vi "Pointer producer consumer Read Voltage.vi"(7 "Total Stop":bool, 8 "error in (no error)":errorcluster, 9 "Speed":u8, 10 "Diodes ON/OFF":bool=TRUE, 11 "Data in":T1={"[V]"=0.0, "Vertical sum"=0.0, "Horizontal sum"=0.0, "auto Loopback"=FALSE, "Auto Balance"=FALSE, "Out Cmd"=0, "Motor Cmd"=0, "ADC Values"=[], "Clouds ctrl"=FALSE, "Cloud Det"=FALSE, "Cloud Sens"=0, "Loops"=0, "VISA res"="COM3"} {"Motor Cmd" format="%x"}) -> (0 "Diods cable OFF status":bool, 1 "Diods cable OFF status request":bool, 2 "ADC votlages":dbl[](array[numeric]), 4 "error out":errorcluster, 5 "Motor Cmd":string=" ")   [LabVIEW 2014]
doc: "INPUTS - baud rate & VISA resource name & convertor selector & motor controler\n\nThis VI sends short HEX number to ATMEGA8 via USB-serial port by NI, and then transform read HEX number into values of convertor Voltage. \n\nOUTPUTS - voltage from ADC0, ADC1, ADC2, ADC3 in ATMEGA8"
uses:
  Ctrls/Data cluster.ctl
panel:
  out "Alfa limit switch":bool
  out "Voltage on ADC0 - UP":dbl format="%#_4g"
  out "Voltage on ADC3 - RIGHT":dbl format="%#_4g"
  out "Voltage on ADC1 - LEFT":dbl format="%#_4g"
  out "Voltage on ADC2 - DOWN":dbl format="%#_4g"
  out "Serial output":string
  out "Serial input":string=" "
  out "VISA resource name":refnum<visa-resource-name>="COM3"
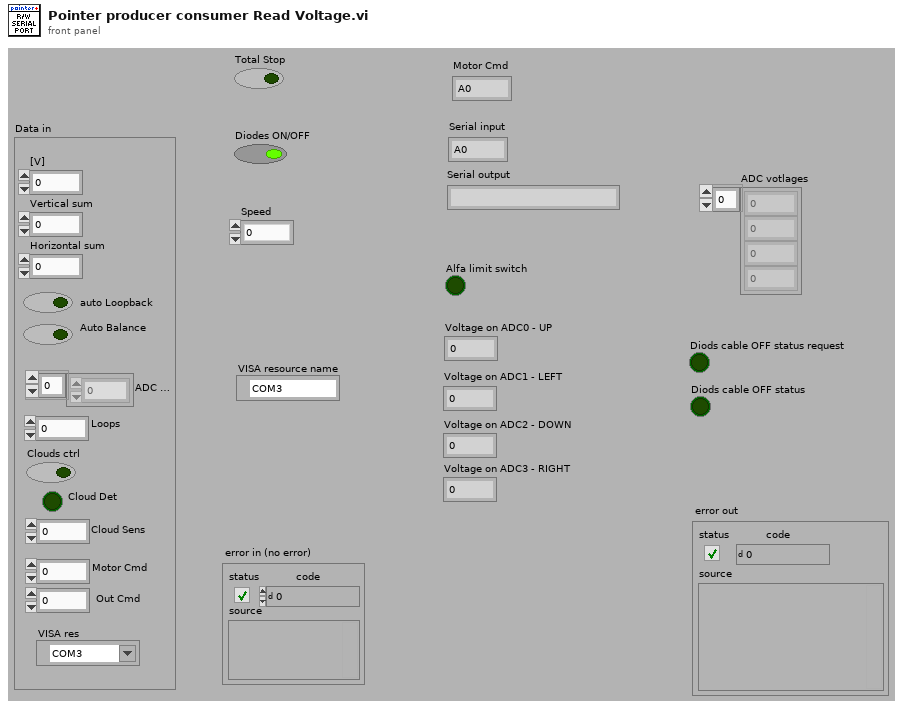
[diagram p1: front panel]
types:
  T1 = typedef "Data cluster.ctl" = cluster{"[V]":dbl, "Vertical sum":dbl, "Horizontal sum":dbl, "auto Loopback":bool, "Auto Balance":bool, "Out Cmd":i32, "Motor Cmd":i32, "ADC Values":dbl[], "Clouds ctrl":bool, "Cloud Det":bool, "Cloud Sens":i8, "Loops":u8, "VISA res":refnum<visa-resource-name>}
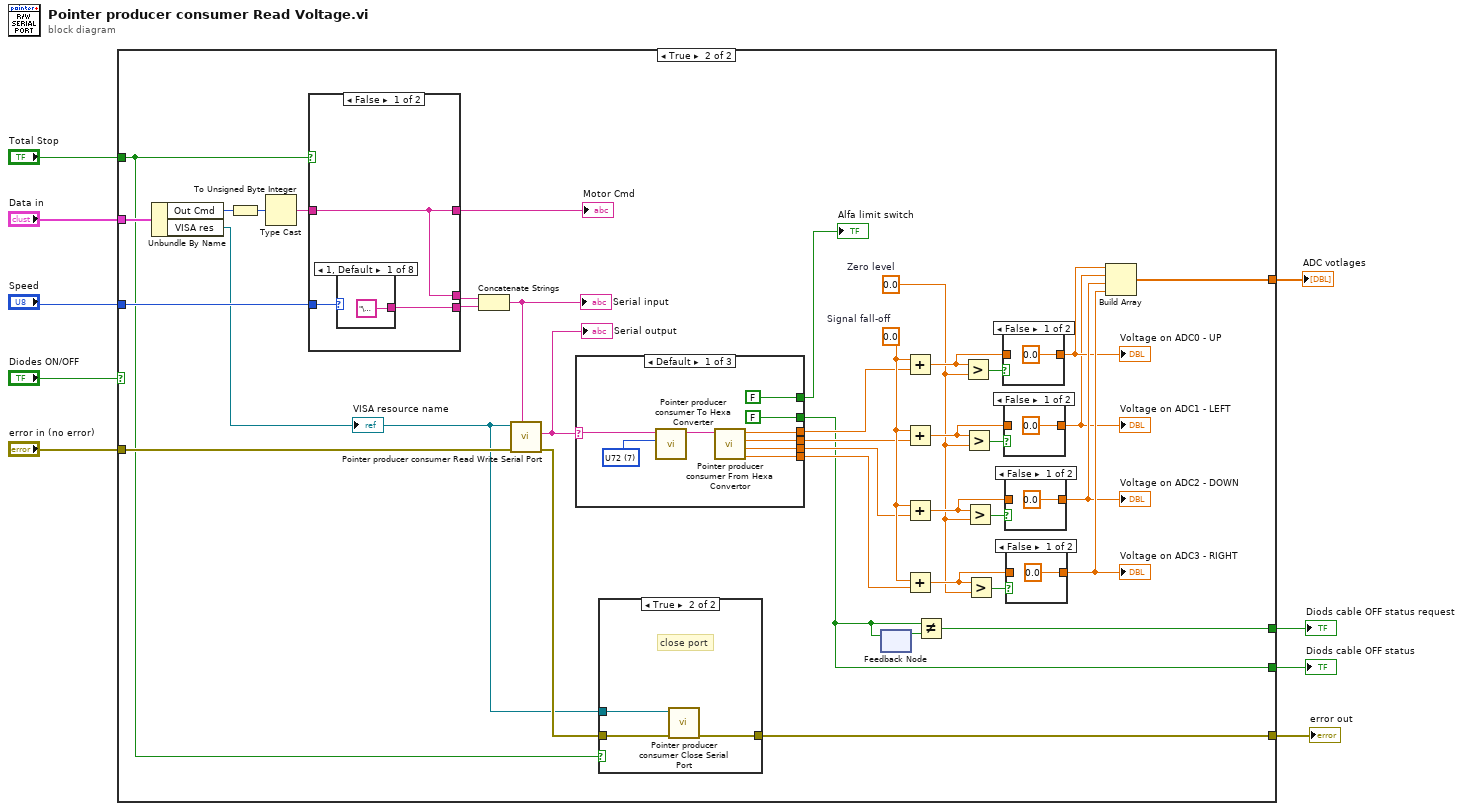
[diagram p0: block diagram]
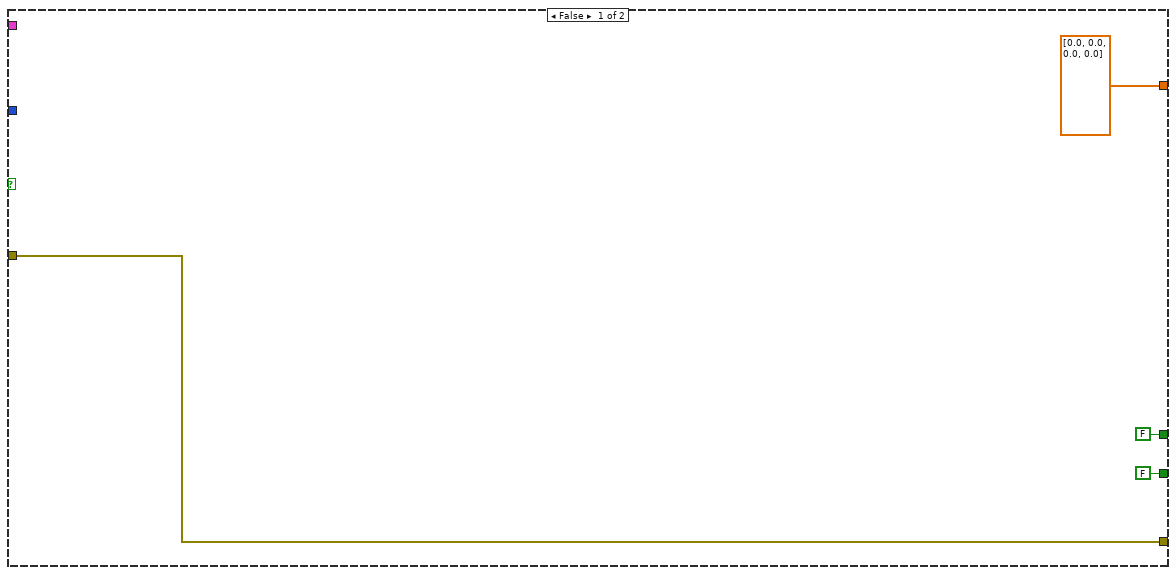
[diagram p2: hidden frame]
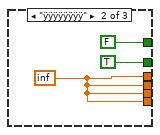
[diagram p4: hidden frame]
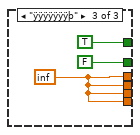
[diagram p5: hidden frame]
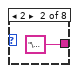
[diagram p10: hidden frame]
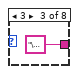
[diagram p11: hidden frame]
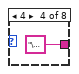
[diagram p12: hidden frame]
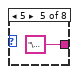
[diagram p13: hidden frame]
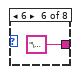
[diagram p14: hidden frame]
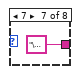
[diagram p15: hidden frame]
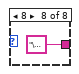
[diagram p16: hidden frame]
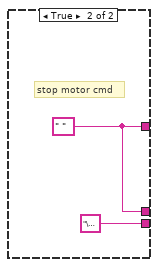
[diagram p17: hidden frame]
diagram:
  n1 = case shown="True" "Diodes ON/OFF" {
    tunnel: [dbl[] [0.0, 0.0, 0.0, 0.0] w27] -> w8
    tunnel: [FALSE w26] -> w7
    tunnel: [FALSE w25] -> w6
    tunnel: "Data in" -> [_ w22]
    tunnel: "Total Stop" -> [_ w15]
    tunnel: "Speed" -> [_ w19]
    tunnel: "error in (no error)" -> [w10 w18]
    tunnel: [w10 w16] -> w1
    frame False {
    }
    frame True {
      w40 = 0.0  # Signal fall-off
      w41 = 0.0  # Zero level
      n2 = Unbundle By Name(w22) -> ("Out Cmd"=w23:i32, "VISA res"=w14:refnum<visa-resource-name>)
      "VISA resource name" <- w14
      n3 = To Unsigned Byte Integer(number=w23) -> (unsigned 8bit integer=w24:u8)
      n4 = Type Cast(x=w24) -> (*(type *) &x=w21:string)  [unwired: 1 in]
      n5 = case shown="False" w15 {
        tunnel: [w79 w90] -> w51
        tunnel: [w80 "\u0000"] -> w50
        tunnel: w19 -> [w81 _]
        tunnel: w21 -> [w79 _]
        tunnel: [w79 w90] -> w20
        frame False {
          n6 = case shown="1, Default" w81 {
            tunnel: ["\u0000" "\u0001" "\u0002" "\u0003" "\u0004" "\u0005" "\u0006" "\u0007"] -> w80
            frame 1, Default {
            }
            frame 2 {
            }
            frame 3 {
            }
            frame 4 {
            }
            frame 5 {
            }
            frame 6 {
            }
            frame 7 {
            }
            frame 8 {
            }
          }
        }
        frame True {
          w90 = " "
          # "stop motor cmd"
        }
      }
      "Motor Cmd" <- w20
      n7 = Concatenate Strings(w51, w50) -> (w28:string)
      "Serial input" <- w28
      n8 = call "Pointer producer consumer Read Write Serial Port.vi"("write string"=w28, "error in (no error)"=w18, "VISA resource name out"=w14) -> ("error out"=w17:errorcluster, "read string"=w29:string)  [unwired: 5 in, 2 out]
      "Serial output" <- w29
      n9 = case shown="Default" w29 {
        selector: w29 -> [w62 _ _]
        tunnel: [w61 w66 w70] -> w39
        tunnel: [w60 w66 w70] -> w38
        tunnel: [w59 w66 w70] -> w37
        tunnel: [w58 w66 w70] -> w36
        tunnel: [FALSE TRUE FALSE] -> w26
        tunnel: [FALSE FALSE TRUE] -> w35
        frame Default {
          w64 = 7 items=["U8", "U16", "U24", "U32", "U48", "U56", "U64", "U72"] ("# Length")
          n10 = call "Pointer producer consumer To Hexa Converter.vi"("# Length"=w64, "NormalIn"=w62) -> ("Normal > Hex"=w63:string)  [unwired: 9 in]
          n11 = call "Pointer producer consumer From Hexa Convertor.vi"("string"=w63) -> ("Voltage on ADC3"=w58:dbl, "Voltage on ADC2"=w59:dbl, "Voltage on ADC1"=w60:dbl, "Voltage on ADC0"=w61:dbl)  [unwired: 7 in]
        }
        frame "ÿÿÿÿÿÿÿÿ" {
          w66 = inf
        }
        frame "ÿÿÿÿÿÿÿþ" {
          w70 = inf
        }
      }
      "Alfa limit switch" <- w35
      n12 = case shown="True" w15 {
        tunnel: w17 -> [w52 w55]
        tunnel: [w52 w54] -> w16
        tunnel: w14 -> [_ w53]
        frame False {
        }
        frame True {
          # "close port"
          n13 = call "Pointer producer consumer Close Serial Port.vi"("error in (no error)"=w55, "VISA resource name"=w53) -> ("error out"=w54:errorcluster)  [unwired: 9 in]
        }
      }
      n14 = feedback #1() -> (w30:bool)  [unwired: 1 in]
      n15 = feedback-in #1(w26) -> ()
      n16 = Add(x=w40, y=w39) -> (x+y=w48:dbl)
      n17 = Add(x=w40, y=w38) -> (x+y=w46:dbl)
      n18 = Add(x=w40, y=w37) -> (x+y=w43:dbl)
      n19 = Add(x=w40, y=w36) -> (x+y=w42:dbl)
      n20 = Not Equal?(x=w26, y=w30) -> (x != y?=w25:bool)
      n21 = Greater?(x=w48, y=w41) -> (0:w49:bool)
      n22 = Greater?(x=w46, y=w41) -> (0:w47:bool)
      n23 = Greater?(x=w43, y=w41) -> (0:w45:bool)
      n24 = Greater?(x=w42, y=w41) -> (0:w44:bool)
      n25 = case shown="False" w49 {
        tunnel: w48 -> [_ w78]
        tunnel: [0.0 w78] -> w32
        frame False {
        }
        frame True {
        }
      }
      "Voltage on ADC0 - UP" <- w32
      n26 = case shown="False" w47 {
        tunnel: w46 -> [_ w76]
        tunnel: [0.0 w76] -> w31
        frame False {
        }
        frame True {
        }
      }
      "Voltage on ADC1 - LEFT" <- w31
      n27 = case shown="False" w45 {
        tunnel: w43 -> [_ w74]
        tunnel: [0.0 w74] -> w33
        frame False {
        }
        frame True {
        }
      }
      "Voltage on ADC2 - DOWN" <- w33
      n28 = case shown="False" w44 {
        tunnel: w42 -> [_ w72]
        tunnel: [0.0 w72] -> w34
        frame False {
        }
        frame True {
        }
      }
      "Voltage on ADC3 - RIGHT" <- w34
      n29 = Build Array(w32, w31, w33, w34) -> (w27:dbl[])
    }
  }
  "ADC votlages" <- w8
  "Diods cable OFF status" <- w7
  "Diods cable OFF status request" <- w6
  "error out" <- w1
